vi "Single Encoder Data.vi"(6 "Reset?":bool, 9 "Tick Constant":dbl, 10 "Rate":dbl, 11 "Distance":dbl) -> (2 "output cluster":T1)   [LabVIEW 2015]
uses:
  <vilib>/addons/control/pid/NI_PID_pid.lvlib
  <vilib>/addons/control/pid/pid.llb/PID Control Input Filter (DBL).vi
panel:
  in  "single encoder cluster":T1
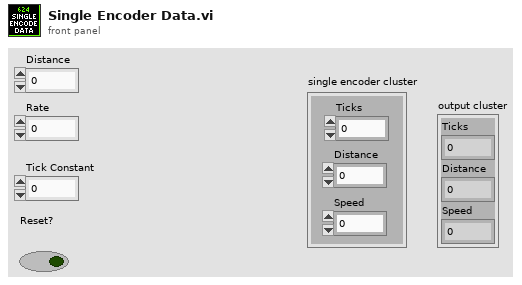
[diagram p1: front panel]
types:
  T1 = cluster{"Ticks":dbl, "Distance":dbl, "Speed":dbl}
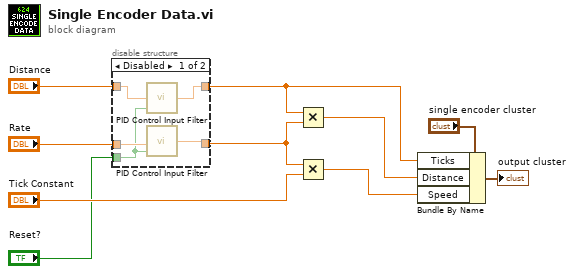
[diagram p0: block diagram]
diagram:
  n1 = disable-structure shown="Disabled" {
    disable-tunnel: "Distance" -> [w15 w17]
    disable-tunnel: "Rate" -> [w13 w16]
    disable-tunnel: [w12 w16] -> w5
    disable-tunnel: [w14 w17] -> w7
    disable-tunnel: "Reset?" -> [w11 _]
    frame Disabled {
      n2 = call-poly <vilib>:"PID Control Input Filter.vi"("reinitialize? (F)"=w11, "input"=w15) -> ("output"=w14:dbl)  [unwired: 3 in]
      n3 = call-poly <vilib>:"PID Control Input Filter.vi"("reinitialize? (F)"=w11, "input"=w13) -> ("output"=w12:dbl)  [unwired: 3 in]
    }
    frame Enabled {
    }
  }
  n4 = Multiply(x=w7, y=w5) -> (x*y=w6:dbl)
  n5 = Multiply(x=w5, y="Tick Constant") -> (x*y=w3:dbl)
  n6 = Bundle By Name(cluster="single encoder cluster", "Ticks"=w7, "Distance"=w6, "Speed"=w3) -> (→"output cluster":T1)
